vi "Construct Target Configuration Command.vi"(8 "error in (no error)":errorcluster, 10 "Target Configuration":T1) -> (0 "error out":errorcluster, 2 "Target Configuration Command":string)   [LabVIEW 2016, in "JLink Commander.lvlib"]
doc: "This VI sends \"-openprj<FILENAME> -open<FILENAME>[,<SADDR>] -auto -exit\" command to JFlash.exe CLI to erase, program and verify the flash. \n\nNote: The parameter Address apply only if the data file is a *.bin file or *.c file."
uses:
  JLink Commander.lvlib
  Type Definitions/Target Configuration.ctl
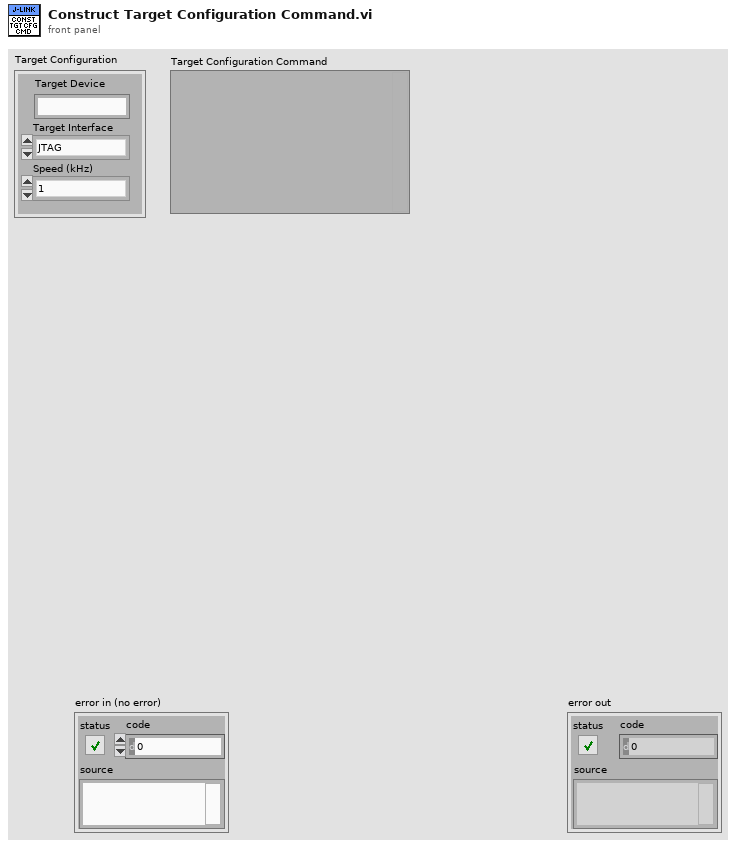
[diagram p1: front panel]
types:
  T1 = typedef "JLink Commander.lvlib/Target Configuration.ctl" = cluster{"Target Device":string, "Target Interface":enum16{"JTAG", "SWD", "FINE", "ICSP", "C2", "CJTAG"}, "Speed (kHz)":enum16{"1", "5", "10", "20", "30", "50", "100", "200", "300", "400", "500", "600", "750", "900", "1000", "1334", "1600", "2000", "2667", "3200", "4000", "4800", "5334", "6000", "8000", "9600", "12000", "15000", "20000", "25000", "30000", "40000", "50000"}}
  T2 = enum16{"JTAG", "SWD", "FINE", "ICSP", "C2", "CJTAG"}
  T3 = enum16{"1", "5", "10", "20", "30", "50", "100", "200", "300", "400", "500", "600", "750", "900", "1000", "1334", "1600", "2000", "2667", "3200", "4000", "4800", "5334", "6000", "8000", "9600", "12000", "15000", "20000", "25000", "30000", "40000", "50000"}
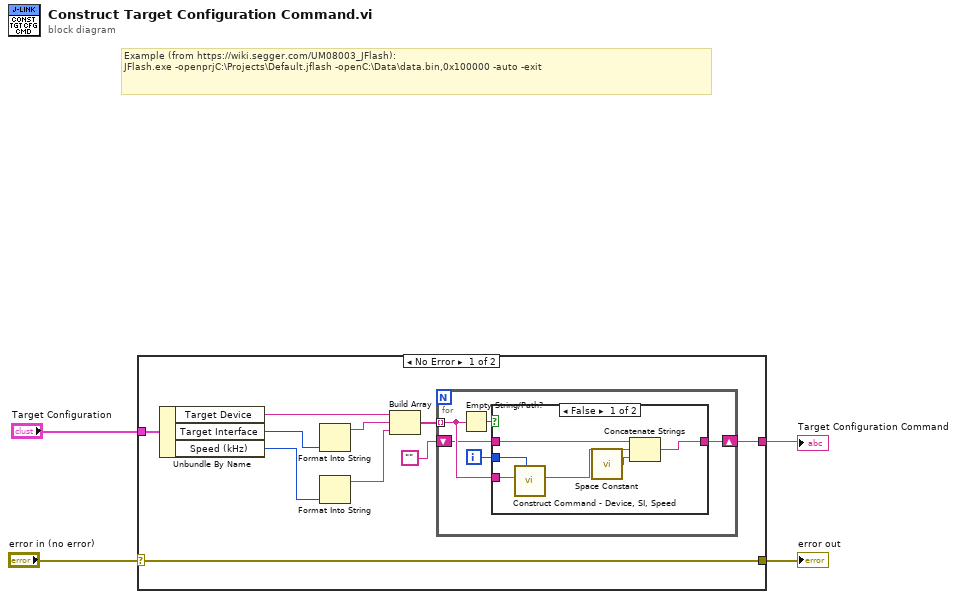
[diagram p0: block diagram]
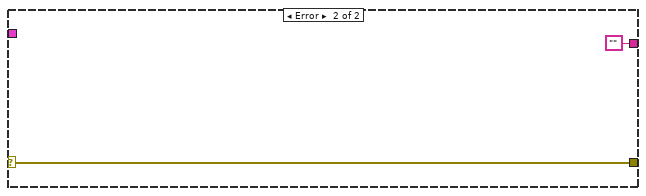
[diagram p3: hidden frame]
diagram:
  # "Example (from https://wiki.segger.com/UM08003_JFlash):\nJFlash.exe -openprjC:\\Projects\\Default.jflash -openC:\\Data\\data.bin,0x100000 -auto -exit"
  n1 = case shown="No Error" "error in (no error)" {
    selector: "error in (no error)" -> [w5 w28]
    tunnel: [w5 w28] -> w3
    tunnel: "Target Configuration" -> [w14 _]
    tunnel: [w6 ""] -> w1
    frame No Error {
      n2 = Unbundle By Name(w14) -> ("Target Device"=w11:string, "Target Interface"=w13:T2, "Speed (kHz)"=w12:T3)
      n3 = Format Into String(w13) -> (resulting string=w10:string)  [unwired: 3 in, 1 out]
      n4 = Format Into String(w12) -> (resulting string=w9:string)  [unwired: 3 in, 1 out]
      n5 = Build Array(w11, w10, w9) -> (w8:string[])
      n6 = for {
        tunnel: w8 -> [w18] mode=indexing
        shift-right: [w16] -> w6
        shift-left: "" -> [w15]
        i -> [w17]
        n7 = Empty String/Path?(string/path=w18) -> (empty?=w19:bool)
        n8 = case shown="False" w19 {
          tunnel: w18 -> [w25 _]
          tunnel: [w22 w26] -> w16
          tunnel: w17 -> [w24 _]
          tunnel: w15 -> [w21 w26]
          frame False {
            n9 = call "Construct Command - Device, SI, Speed.vi"("Configuration Type"=w24, "Input"=w25) -> ("Output"=w23:string)  [unwired: 8 in, 1 out]
            n10 = call <vilib>:"Space Constant.vi"() -> ("String"=w20:string)
            n11 = Concatenate Strings(w21, w23, w20) -> (w22:string)
          }
          frame True {
          }
        }
      }
    }
    frame Error {
    }
  }
  "error out" <- w3
  "Target Configuration Command" <- w1
